vi "488.vi"() -> ()   [LabVIEW 2025]
panel:
  out "equipo":string[](array[string])
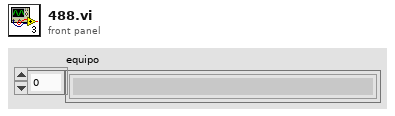
[diagram p1: front panel]
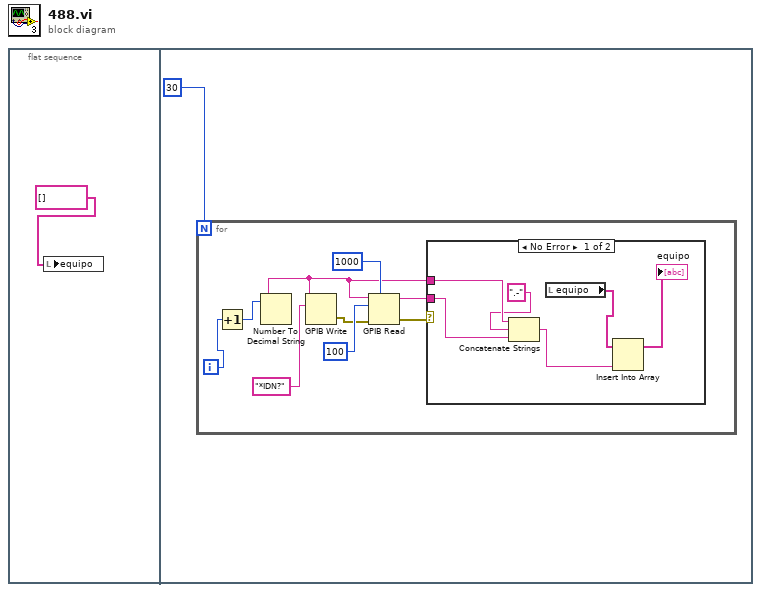
[diagram p0: block diagram]
diagram:
  n1 = flat-sequence {
    frame #0 {
      n2 = local write "equipo"(string[] []) -> ()
    }
    frame #1 {
      n3 = for {
        N: 30 -> [_]
        i -> [w11]
        n4 = Increment(x=w11) -> (x+1=w10:i32)
        n5 = Number To Decimal String(number=w10) -> (decimal integer string=w5:string)  [unwired: 1 in]
        n6 = GPIB Write(0:w5, 1:"*IDN?") -> (6:w7:errorcluster)  [unwired: 3 in, 1 out]
        n7 = GPIB Read(0:w5, 1:100, 3:w7, 4:1000) -> (5:w4:string, 7:w3:errorcluster)  [unwired: 1 in, 1 out]
        n8 = case shown="No Error" w3 {
          tunnel: w5 -> [w17 _]
          tunnel: w4 -> [w16 _]
          frame No Error {
            n9 = Concatenate Strings(w17, ".-", w16) -> (w14:string)
            n10 = local read "equipo"() -> (w12:string[])
            n11 = Insert Into Array(array=w12, new element=w14) -> (→"equipo":string[])  [unwired: 1 in]
          }
          frame Error {
          }
        }
      }
    }
  }
